vi "Get String Error Contexts.vi"(9 "index of error":i32, 10 "expected string":string, 11 "actual string":string) -> (1 "Actual Context":string, 2 "expected char":string, 3 "actual char":string)   [LabVIEW 2015, in "VITAC.lvlib"]
uses:
  VITAC.lvlib
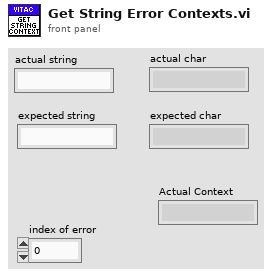
[diagram p1: front panel]
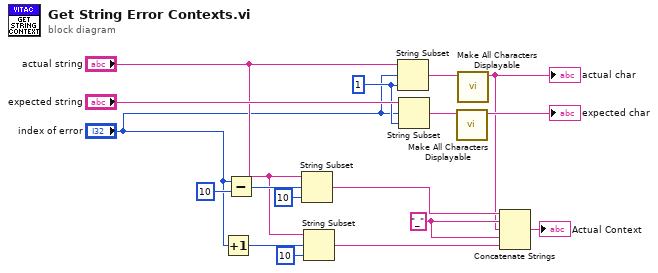
[diagram p0: block diagram]
diagram:
  w5 = "_" ("string")
  w15 = 1 ("length")
  n1 = Increment(x="index of error") -> (x+1=w7:i32)
  n2 = Subtract(x="index of error", y=10) -> (x-y=w12:i32)
  n3 = String Subset(string="actual string", offset (0)=w12, length (rest)=10 ("length (rest)")) -> (substring=w6:string)
  n4 = String Subset(string="actual string", offset (0)=w7, length (rest)=10 ("length (rest)")) -> (substring=w4:string)
  n5 = String Subset(string="actual string", offset (0)="index of error", length (rest)=w15) -> (substring=w3:string)
  n6 = String Subset(string="expected string", offset (0)="index of error", length (rest)=w15) -> (substring=w16:string)
  n7 = call "Make All Characters Displayable.vi"("String In"=w16) -> ("Escaped String"=→"expected char":string)  [unwired: 10 in]
  n8 = call "Make All Characters Displayable.vi"("String In"=w3) -> ("Escaped String"=w1:string)  [unwired: 10 in]
  "actual char" <- w1
  n9 = Concatenate Strings(w6, w5, w1, w5, w4) -> (→"Actual Context":string)
